vi "Parameters.vi"(8 "error in (no error)":errorcluster, 11 "Template Test Case In":refnum<class "String Parser Test.lvclass">) -> (0 "error out":errorcluster, 2 "Parameters":T1(array[cluster]))   [LabVIEW 2020, in "String Parser Test.lvclass"]
uses:
  String Parser Test.lvclass
  C:/Users/SAS/Desktop/astemes-lunit-parameterized-test/source/Parameterized Test Case/Parameterized Test Case.lvclass
  source/Parameterized Test Case/Parameterized Test Case.lvclass
  String Parser Test.lvclass/String Parser Test.ctl
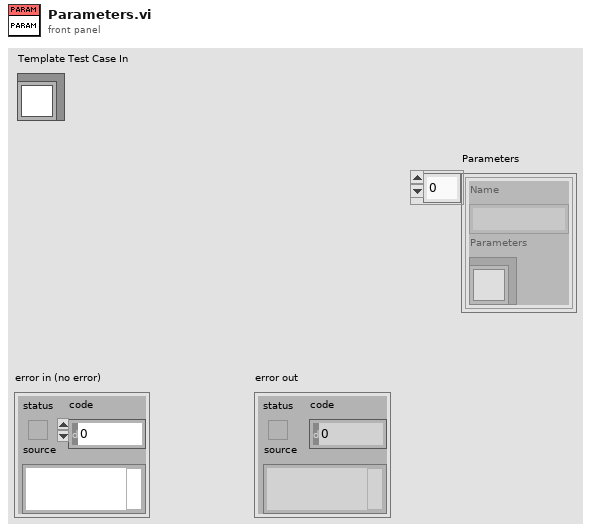
[diagram p1: front panel]
types:
  T1 = cluster{"Name":string, "Parameters":refnum<class "Parameterized Test Case.lvclass">}[]
  T2 = cluster{"Name":string, "String Parser Test.lvclass":refnum<class "String Parser Test.lvclass">}
  T3 = cluster{"Name":string, "String Parser Test.lvclass":refnum<class "String Parser Test.lvclass">}[]
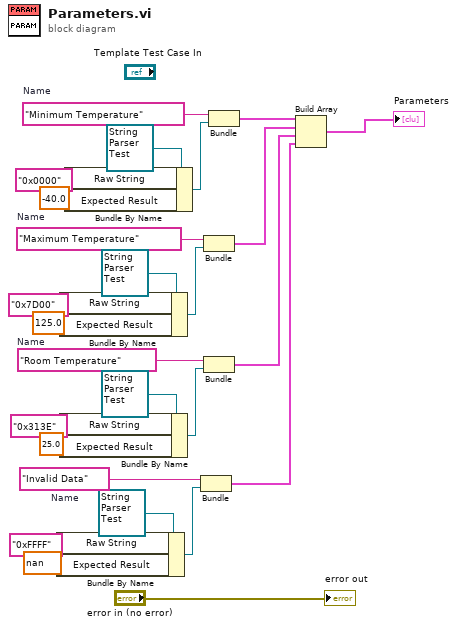
[diagram p0: block diagram]
diagram:
  w2 = "Invalid Data"  # Name
  w13 = "Room Temperature"  # Name
  w14 = "Maximum Temperature"  # Name
  w25 = "Minimum Temperature"  # Name
  n1 = Bundle By Name(cluster=refnum<class "String Parser Test.lvclass"> refnum ("String Parser Test.lvclass"), "Raw String"="0xFFFF", "Expected Result"=nan) -> (w4:refnum<class "String Parser Test.lvclass">)
  n2 = Bundle By Name(cluster=refnum<class "String Parser Test.lvclass"> refnum ("String Parser Test.lvclass"), "Raw String"="0x7D00", "Expected Result"=125.0) -> (w16:refnum<class "String Parser Test.lvclass">)
  n3 = Bundle By Name(cluster=refnum<class "String Parser Test.lvclass"> refnum ("String Parser Test.lvclass"), "Raw String"="0x313E", "Expected Result"=25.0) -> (w11:refnum<class "String Parser Test.lvclass">)
  n4 = Bundle By Name(cluster=refnum<class "String Parser Test.lvclass"> refnum ("String Parser Test.lvclass"), "Raw String"="0x0000", "Expected Result"=-40.0) -> (w23:refnum<class "String Parser Test.lvclass">)
  n5 = Bundle "Bundle"("Name"=w2, "String Parser Test.lvclass"=w4) -> (w1:T2)  [unwired: 1 in]
  n6 = Bundle "Bundle"("Name"=w14, "String Parser Test.lvclass"=w16) -> (w8:T2)  [unwired: 1 in]
  n7 = Bundle "Bundle"("Name"=w13, "String Parser Test.lvclass"=w11) -> (w7:T2)  [unwired: 1 in]
  n8 = Bundle "Bundle"("Name"=w25, "String Parser Test.lvclass"=w23) -> (w20:T2)  [unwired: 1 in]
  n9 = Build Array "Build Array"(w20, w8, w7, w1) -> (→"Parameters":T3)
  "error out" <- "error in (no error)"
